vi "Clear Bookmarks.vi"(8 "Error In":errorcluster, 11 "State In":T1) -> (0 "Error Out":errorcluster, 3 "State Out":T1)   [LabVIEW 2017, in "Bookmark Manager.lvlib"]
uses:
  Bookmark Manager.lvlib
  State.ctl
  VI Bookmark.ctl
  VI Information.ctl
  Application Information.ctl
  Bookmarks Views.ctl
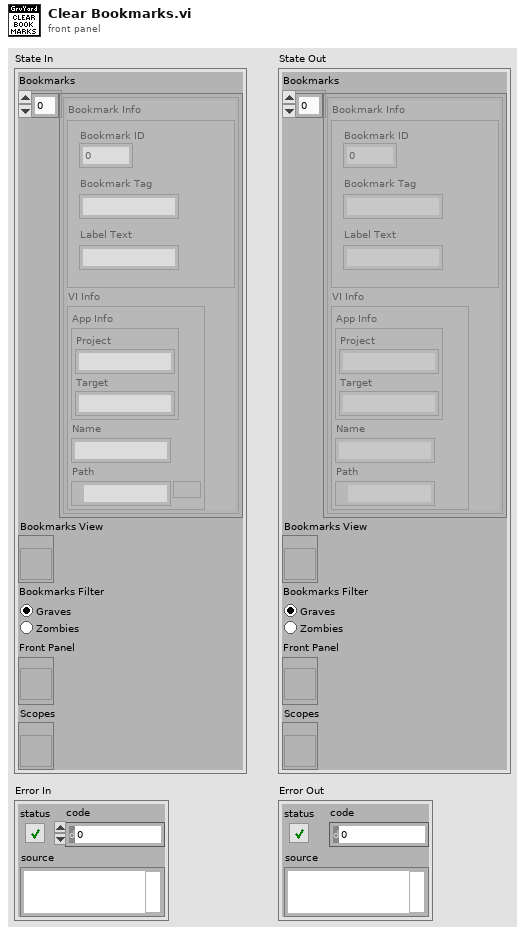
[diagram p1: front panel]
types:
  T1 = typedef "Bookmark Manager.lvlib/State.ctl" = cluster{"Bookmarks":T2[], "Bookmarks View":refnum<vi>, "Bookmarks Filter":T5, "Front Panel":refnum<vi>, "Scopes":refnum<vi>}
  T2 = typedef "Bookmark Manager.lvlib/VI Bookmark.ctl" = cluster{"Bookmark Info":cluster{"Bookmark ID":u32, "Bookmark Tag":string, "Label Text":string}, "VI Info":T3}
  T3 = typedef "Bookmark Manager.lvlib/VI Information.ctl" = cluster{"App Info":T4, "Name":string, "Path":path}
  T4 = typedef "Bookmark Manager.lvlib/Application Information.ctl" = cluster{"Project":string, "Target":string}
  T5 = typedef "Bookmark Manager.lvlib/Bookmarks Views.ctl" = enum32{"Graves", "Zombies"}
  T6 = enum8{"Enabled", "Disabled", "Disabled and Grayed Out"}
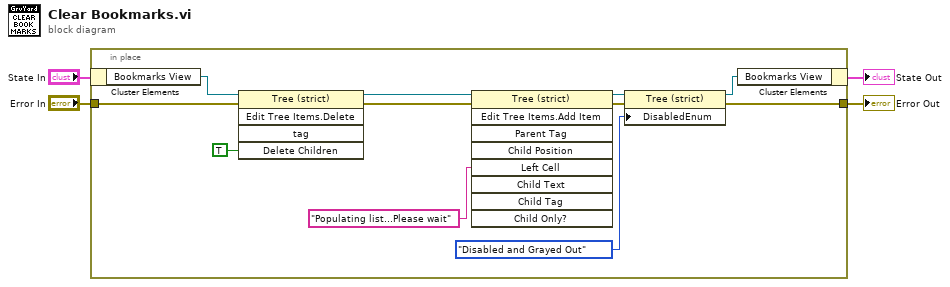
[diagram p0: block diagram]
diagram:
  n1 = in-place {
    in-place-border: "Error In" -> [w6]
    in-place-border: [w5] -> w4
    n2 = in-place-cluster #1("State In") -> ("Bookmarks View"=w8:refnum<vi>)
    n3 = invoke class="Tree (strict)" method="Edit Tree Items.Delete"(reference=w8, error in=w6, "Delete Children"=TRUE ("Delete Children?")) -> (reference out=w14:refnum<vi>, error out=w13:errorcluster)  [unwired: 2 in, 3 out]
    n4 = invoke class="Tree (strict)" method="Edit Tree Items.Add Item"(reference=w14, error in=w13, "Left Cell"="Populating list...Please wait" ("Left Cell String")) -> (reference out=w11:refnum<vi>, error out=w10:errorcluster)  [unwired: 6 in, 7 out]
    n5 = property class="Tree (strict)"(reference=w11, error in=w10, "DisabledEnum"=T6."Disabled and Grayed Out" ("Disabled")) -> (reference out=w7:refnum<vi>, error out=w5:errorcluster)
    n6 = in-place-cluster #1("Bookmarks View"=w7) -> (→"State Out":T1)
  }
  "Error Out" <- w4
